vi "SVT Initialize Swept Sine (DAQmx) (1 AO, 2 AI).vi"(8 "error in (no error)":errorcluster, 9 "AI response settings":T5={"response channel"="", "max value [V]"=10.0, "min value [V]"=-10.0, "terminal configuration"=-1} {"terminal configuration" items=["Default"=-1, "RSE"=10083, "NRSE"=10078, "Differential"=10106, "Pseudodifferential"=12529]; "min value [V]" format="%.2f"; "max value [V]" format="%.2f"}, 10 "AI stimulus settings":T6={"stimulus channel"="", "max value [V]"=10.0, "min value [V]"=-10.0, "terminal configuration"=-1} {"terminal configuration" items=["Default"=-1, "RSE"=10083, "NRSE"=10078, "Differential"=10106, "Pseudodifferential"=12529]; "min value [V]" format="%.2f"; "max value [V]" format="%.2f"}, 11 "AO source settings":T7={"excitation channel"="", "max value [V]"=10.0, "min value [V]"=-10.0, "terminal configuration"=-1} {"terminal configuration" items=["Default"=-1, "RSE"=10083, "Differential"=10106, "Pseudodifferential"=12529]; "min value [V]" format="%0.2f"; "max value [V]" format="%0.2f"}) -> (0 "error out":errorcluster, 3 "swept sine task out":T1={"source settings"={"AO task name"="", "source"=[]}, "stimulus settings"={"stimulus task name"="", "stimulus"=[]}, "response(s) settings"={"response task name"="", "response"=[]}, "measurement settings"={"AI sampling frequency"=51200.0, "AO sampling frequency"=1024.0, "AI block size"=1024, "AO block Size"=1024, "block duration [ms]"=0.0, "number of AI channels"=0, "device propagation delay [samples]"=0.0, "total propagation time [samples]"=0.0, "DUT propagation time [ms]"=0.0}, "linlog"=enum."linear", "repeat"=enum."off", "frequency list"=[1.0], "amplitude list"=[1.0], "settling time"={"settle time"=0.015599999576807022, "settle cycles"=5}, "integration time"={"integration time"=0.015599999576807022, "integration cycles"=5}, "frequencies indices"={"AI freq index"=0, "AO freq index"=5}, "read marks"={"write index"=0, "read index"=0, "freq start index"=0, "freq stop index"=0, "# extracted"=0, "buffer type"=enum."Invalid buffer", "read/write indices"=[], "AO index"=0, "AI index"=0, "settled"=FALSE, "integration done"=FALSE}, "harmonic settings"={"maximum THD harmonic"=5, "harmonic mapping"=[1], "units"={"THD unit"=enum."%", "nth harmonic unit"=enum."%", "SINAD unit"=enum."dB", "THD+N unit"=enum."dB"}}, "auto resolution settings"={"auto max step"=512, "slow threshold db"=6.0, "fast threshold db"=1.0}, "auto level settings"={"auto level enable"=FALSE, "auto level channel"=6, "ideal ref"=1.0, "max level"=10.0, "ref upper deviation db"=3.0, "ref lower deviation db"=-3.0}, "offset"=1.0, "ramping rate"=0.0, "phase"=0.0, "initialize"=FALSE} {"phase" format="%.2f"; "response(s) settings"."response"."channel info"."pregain" format="%.2f"; "response(s) settings"."response"."channel info"."weighting filter" items=["Linear", "A-weighting", "B-weighting", "C-weighting", "ITU-R 468-4", "Dolby", "CCITT", "C-message", "Wb", "Wc", "Wd", "We", "Wf", "Wh", "Wj", "Wk", "Wm", "AES17 20 kHz lowpass", "AES17 40 kHz lowpass", "AES17 20 kHz highpass", "AES17 40 kHz highpass"]; "response(s) settings"."response"."channel info"."dB reference" format="%^.1e"; "response(s) settings"."response"."channel info"."engineering units" items=["custom..."=0, "V"=1, "A"=21, "C"=30, "pC"=31, "s"=32, "-"=29, "Pa"=2, "N"=20, "g"=3, "m/s^2"=4, "m/s"=5, "m"=6, "mm/s"=12, "mm"=13, "micron/s"=14, "micron"=15, "in/s^2"=7, "in/s"=8, "in"=9, "mil/s"=10, "mil"=11, "rad/s^2"=16, "rad/s"=17, "rad"=18, "deg/s^2"=26, "deg/s"=27, "deg"=28, "RPM"=22, "cycle/s^2"=23, "Hz"=24, "cycle"=25, "strain"=19]; "response(s) settings"."response"."channel info"."sensor sensitivity" format="%#_5f"; "stimulus settings"."stimulus"."channel info"."pregain" format="%.2f"; "stimulus settings"."stimulus"."channel info"."weighting filter" items=["Linear", "A-weighting", "B-weighting", "C-weighting", "ITU-R 468-4", "Dolby", "CCITT", "C-message", "Wb", "Wc", "Wd", "We", "Wf", "Wh", "Wj", "Wk", "Wm", "AES17 20 kHz lowpass", "AES17 40 kHz lowpass", "AES17 20 kHz highpass", "AES17 40 kHz highpass"]; "stimulus settings"."stimulus"."channel info"."dB reference" format="%^.1e"; "stimulus settings"."stimulus"."channel info"."engineering units" items=["custom..."=0, "V"=1, "A"=21, "C"=30, "pC"=31, "s"=32, "-"=29, "Pa"=2, "N"=20, "g"=3, "m/s^2"=4, "m/s"=5, "m"=6, "mm/s"=12, "mm"=13, "micron/s"=14, "micron"=15, "in/s^2"=7, "in/s"=8, "in"=9, "mil/s"=10, "mil"=11, "rad/s^2"=16, "rad/s"=17, "rad"=18, "deg/s^2"=26, "deg/s"=27, "deg"=28, "RPM"=22, "cycle/s^2"=23, "Hz"=24, "cycle"=25, "strain"=19]; "stimulus settings"."stimulus"."channel info"."sensor sensitivity" format="%#_5f"; "ramping rate" format="%.4f"; "offset" format="%.2f"; "auto level settings"."ref lower deviation db" format="%.4f"; "auto level settings"."ref upper deviation db" format="%.4f"; "auto level settings"."max level" format="%.4f"; "auto level settings"."ideal ref" format="%.4f"; "auto resolution settings"."fast threshold db" format="%.4f"; "auto resolution settings"."slow threshold db" format="%.4f"; "harmonic settings"."maximum THD harmonic" max=10 step=1; "integration time"."integration time" format="%.2p"; "settling time"."settle time" format="%.2p"; "amplitude list" format="%.2f"; "frequency list" format="%.2f"; "measurement settings"."DUT propagation time [ms]" format="%.2f"; "measurement settings"."AO sampling frequency" format="%.2f"; "measurement settings"."AI sampling frequency" format="%.2f"})   [LabVIEW 2017, in "SoundVib_SweptSine.lvlib"]
doc: "Initializes swept-sine-analysis parameters on analog input and output devices."
uses:
  <vilib>/addons/Sound and Vibration/svt_Swept Sine/SoundVib_SweptSine.lvlib
  <vilib>/addons/Sound and Vibration/svt_Swept Sine/subVIs/sv_Swept Sine Task.ctl
  <vilib>/addons/_NISVFA/_Shared subVIs/Controls/svc_Channel Info.ctl
  <vilib>/addons/_NISVFA/_Shared subVIs/Controls/svc_Engineering Units Text Ring.ctl
  <vilib>/addons/_NISVFA/_Shared subVIs/Controls/svc_Weighting Filter Text Ring.ctl
  <vilib>/DAQmx/create/channels.llb/DAQmx Create Channel (AI-Voltage-Basic).vi
  <vilib>/DAQmx/create/channels.llb/DAQmx Create Channel (AO-Voltage-Basic).vi
  <resource>/objmgr/daqmx.rc
panel:
  in  "swept sine task default":T1={"source settings"={"AO task name"="", "source"=[]}, "stimulus settings"={"stimulus task name"="", "stimulus"=[]}, "response(s) settings"={"response task name"="", "response"=[]}, "measurement settings"={"AI sampling frequency"=51200.0, "AO sampling frequency"=51200.0, "AI block size"=1024, "AO block Size"=0, "block duration [ms]"=1024.0, "number of AI channels"=0, "device propagation delay [samples]"=0.0, "total propagation time [samples]"=0.0, "DUT propagation time [ms]"=0.0}, "linlog"=enum."linear", "repeat"=enum."off", "frequency list"=[1.0], "amplitude list"=[1.0], "settling time"={"settle time"=0.015599999576807022, "settle cycles"=5}, "integration time"={"integration time"=0.015599999576807022, "integration cycles"=5}, "frequencies indices"={"AI freq index"=0, "AO freq index"=0}, "read marks"={"write index"=0, "read index"=0, "freq start index"=0, "freq stop index"=0, "# extracted"=0, "buffer type"=enum."Invalid buffer", "read/write indices"=[], "AO index"=0, "AI index"=0, "settled"=FALSE, "integration done"=FALSE}, "harmonic settings"={"maximum THD harmonic"=5, "harmonic mapping"=[1], "units"={"THD unit"=enum."%", "nth harmonic unit"=enum."%", "SINAD unit"=enum."dB", "THD+N unit"=enum."dB"}}, "auto resolution settings"={"auto max step"=512, "slow threshold db"=6.0, "fast threshold db"=1.0}, "auto level settings"={"auto level enable"=FALSE, "auto level channel"=0, "ideal ref"=1.0, "max level"=10.0, "ref upper deviation db"=3.0, "ref lower deviation db"=-3.0}, "offset"=1.0, "ramping rate"=0.0, "phase"=0.0, "initialize"=FALSE} {"phase" format="%.2f"; "response(s) settings"."response"."channel info"."pregain" format="%.2f"; "response(s) settings"."response"."channel info"."weighting filter" items=["Linear", "A-weighting", "B-weighting", "C-weighting", "ITU-R 468-4", "Dolby", "CCITT", "C-message", "Wb", "Wc", "Wd", "We", "Wf", "Wh", "Wj", "Wk", "Wm", "AES17 20 kHz lowpass", "AES17 40 kHz lowpass", "AES17 20 kHz highpass", "AES17 40 kHz highpass"]; "response(s) settings"."response"."channel info"."dB reference" format="%^.1e"; "response(s) settings"."response"."channel info"."engineering units" items=["custom..."=0, "V"=1, "A"=21, "C"=30, "pC"=31, "s"=32, "-"=29, "Pa"=2, "N"=20, "g"=3, "m/s^2"=4, "m/s"=5, "m"=6, "mm/s"=12, "mm"=13, "micron/s"=14, "micron"=15, "in/s^2"=7, "in/s"=8, "in"=9, "mil/s"=10, "mil"=11, "rad/s^2"=16, "rad/s"=17, "rad"=18, "deg/s^2"=26, "deg/s"=27, "deg"=28, "RPM"=22, "cycle/s^2"=23, "Hz"=24, "cycle"=25, "strain"=19]; "response(s) settings"."response"."channel info"."sensor sensitivity" format="%#_5f"; "stimulus settings"."stimulus"."channel info"."pregain" format="%.2f"; "stimulus settings"."stimulus"."channel info"."weighting filter" items=["Linear", "A-weighting", "B-weighting", "C-weighting", "ITU-R 468-4", "Dolby", "CCITT", "C-message", "Wb", "Wc", "Wd", "We", "Wf", "Wh", "Wj", "Wk", "Wm", "AES17 20 kHz lowpass", "AES17 40 kHz lowpass", "AES17 20 kHz highpass", "AES17 40 kHz highpass"]; "stimulus settings"."stimulus"."channel info"."dB reference" format="%^.1e"; "stimulus settings"."stimulus"."channel info"."engineering units" items=["custom..."=0, "V"=1, "A"=21, "C"=30, "pC"=31, "s"=32, "-"=29, "Pa"=2, "N"=20, "g"=3, "m/s^2"=4, "m/s"=5, "m"=6, "mm/s"=12, "mm"=13, "micron/s"=14, "micron"=15, "in/s^2"=7, "in/s"=8, "in"=9, "mil/s"=10, "mil"=11, "rad/s^2"=16, "rad/s"=17, "rad"=18, "deg/s^2"=26, "deg/s"=27, "deg"=28, "RPM"=22, "cycle/s^2"=23, "Hz"=24, "cycle"=25, "strain"=19]; "stimulus settings"."stimulus"."channel info"."sensor sensitivity" format="%#_5f"; "ramping rate" format="%.4f"; "offset" format="%.2f"; "auto level settings"."ref lower deviation db" format="%.4f"; "auto level settings"."ref upper deviation db" format="%.4f"; "auto level settings"."max level" format="%.4f"; "auto level settings"."ideal ref" format="%.4f"; "auto resolution settings"."fast threshold db" format="%.4f"; "auto resolution settings"."slow threshold db" format="%.4f"; "harmonic settings"."maximum THD harmonic" max=10 step=1; "integration time"."integration time" format="%.2p"; "settling time"."settle time" format="%.2p"; "amplitude list" format="%.2f"; "frequency list" format="%.2f"; "measurement settings"."DUT propagation time [ms]" format="%.2f"; "measurement settings"."AO sampling frequency" format="%.2f"; "measurement settings"."AI sampling frequency" format="%.2f"}
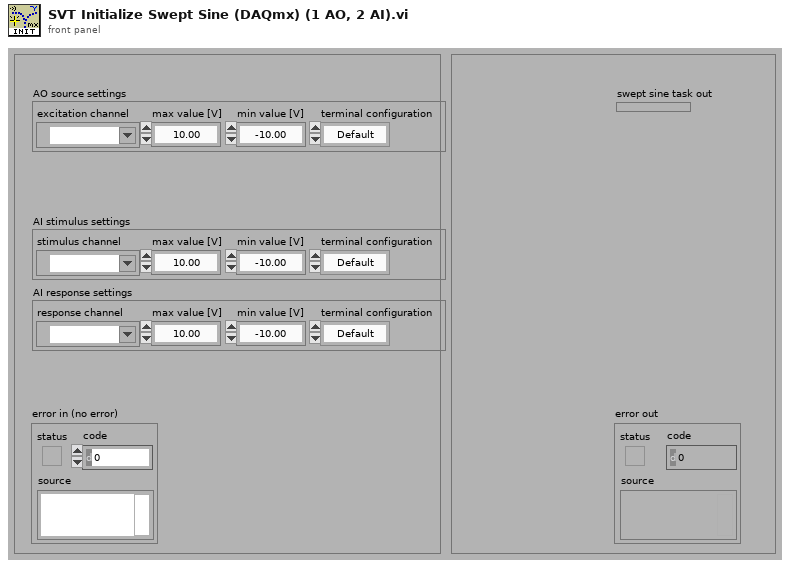
[diagram p1: front panel]
types:
  T1 = typedef "SoundVib_SweptSine.lvlib/sv_Swept Sine Task.ctl" = cluster{"source settings":cluster{"AO task name":refnum<k21>, "source":cluster{"AO physical channel":tag}[]}, "stimulus settings":cluster{"stimulus task name":refnum<k21>, "stimulus":cluster{"stimulus physical channel":tag, "channel info":T2}[]}, "response(s) settings":cluster{"response task name":refnum<k21>, "response":cluster{"response physical channel":tag, "channel info":T2}[]}, "measurement settings":cluster{"AI sampling frequency":dbl, "AO sampling frequency":dbl, "AI block size":i32, "AO block Size":i32, "block duration [ms]":dbl, "number of AI channels":i32, "device propagation delay [samples]":dbl, "total propagation time [samples]":dbl, "DUT propagation time [ms]":dbl}, "linlog":enum16{"linear", "log"}, "repeat":enum16{"off", "on"}, "frequency list":dbl[], "amplitude list":dbl[], "settling time":cluster{"settle time":dbl, "settle cycles":i32}, "integration time":cluster{"integration time":dbl, "integration cycles":i32}, "frequencies indices":cluster{"AI freq index":i32, "AO freq index":i32}, "read marks":cluster{"write index":u32, "read index":u32, "freq start index":u32, "freq stop index":u32, "# extracted":u32, "buffer type":enum16{"Invalid buffer", "Intermediate buffer", "Final buffer"}, "read/write indices":cluster{"settle time index":u32, "integration time index":u32}[], "AO index":i32, "AI index":i32, "settled":bool, "integration done":bool}, "harmonic settings":cluster{"maximum THD harmonic":u32, "harmonic mapping":u32[], "units":cluster{"THD unit":enum16{"dB", "%"}, "nth harmonic unit":enum16{"dB", "%"}, "SINAD unit":enum16{"dB", "%"}, "THD+N unit":enum16{"dB", "%"}}}, "auto resolution settings":cluster{"auto max step":i32, "slow threshold db":dbl, "fast threshold db":dbl}, "auto level settings":cluster{"auto level enable":bool, "auto level channel":u8, "ideal ref":sgl, "max level":sgl, "ref upper deviation db":sgl, "ref lower deviation db":sgl}, "offset":dbl, "ramping rate":dbl, "phase":dbl, "initialize":bool}
  T2 = typedef "svc_Channel Info.ctl" = cluster{"sensor sensitivity":dbl, "engineering units":T3, "dB reference":dbl, "custom label":string, "weighting filter":T4, "pregain":dbl}
  T3 = typedef "svc_Engineering Units Text Ring.ctl" = u16
  T4 = typedef "svc_Weighting Filter Text Ring.ctl" = u16
  T5 = cluster{"response channel":tag, "max value [V]":dbl, "min value [V]":dbl, "terminal configuration":i32}
  T6 = cluster{"stimulus channel":tag, "max value [V]":dbl, "min value [V]":dbl, "terminal configuration":i32}
  T7 = cluster{"excitation channel":tag, "max value [V]":dbl, "min value [V]":dbl, "terminal configuration":i32}
  T8 = cluster{"settle time index":u32, "integration time index":u32}[]
  T9 = enum16{"Invalid buffer", "Intermediate buffer", "Final buffer"}
  T10 = cluster{"DAQmx Physical Channel":tag, "channel info":T2}
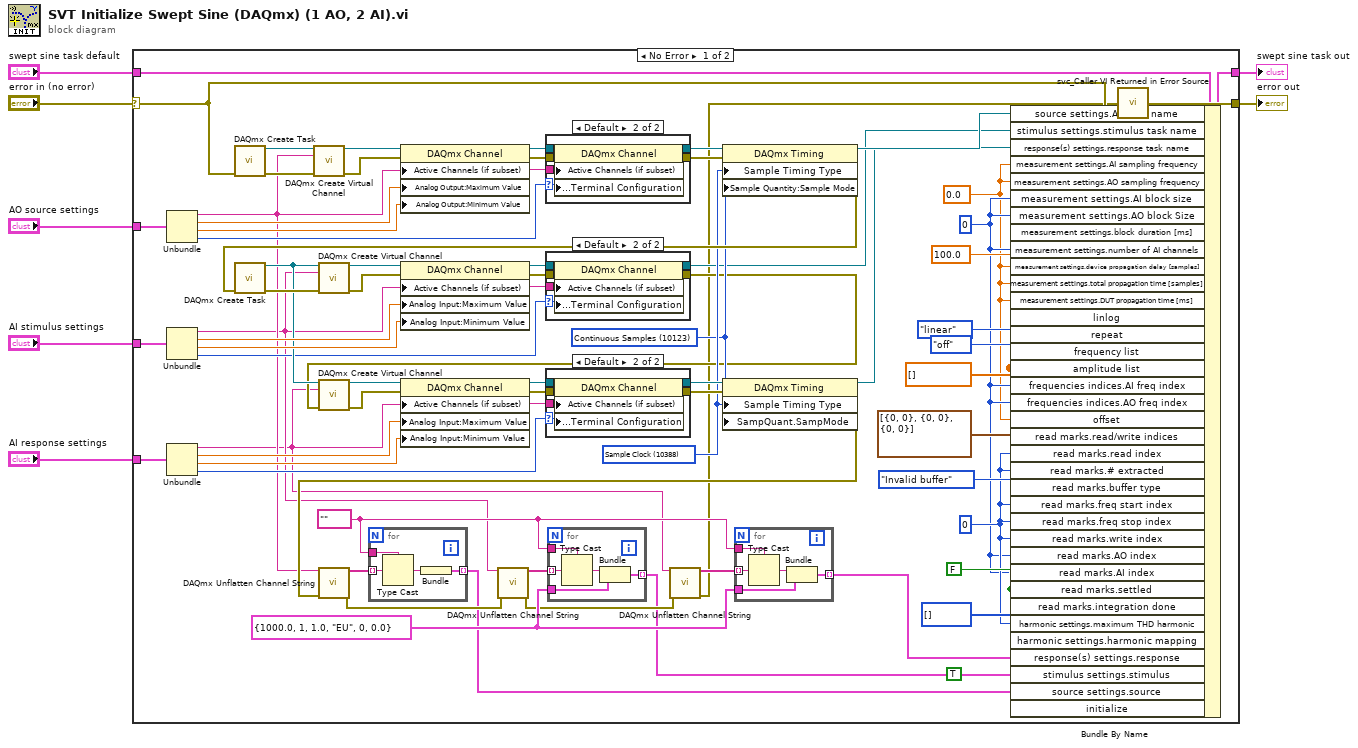
[diagram p0: block diagram]
diagram:
  n1 = case shown="No Error" "error in (no error)" {
    selector: "error in (no error)" -> [w15 w117]
    tunnel: [w70 w117] -> w6
    tunnel: [w67 w116] -> w5
    tunnel: "AO source settings" -> [w55 _]
    tunnel: "AI stimulus settings" -> [w62 _]
    tunnel: "AI response settings" -> [w58 _]
    tunnel: "swept sine task default" -> [w69 w116]
    frame No Error {
      w46 = T2 {"sensor sensitivity"=1000.0, "engineering units"=1, "dB reference"=1.0, "custom label"="EU", "weighting filter"=0, "pregain"=0.0} ("channel info")
      w75 = dbl[] [] ("frequency list")
      w35 = 0.0 ("measurement settings.AI sampling frequency")
      w14 = 10123 items=["Finite Samples"=10178, "Continuous Samples"=10123, "Hardware Timed Single Point"=12522] ("SampQuant.SampMode")
      w17 = 10388 items=["Sample Clock"=10388, "Handshake"=10389, "Implicit"=10451, "On Demand"=10390, "Change Detection"=12504] ("SampTimingType")
      w39 = 0 ("AO device settings.AO Settings.AO taskID")
      w43 = tag "" ("DAQmx Physical Channel")
      w73 = FALSE ("acq state.settled")
      w68 = u32 0 ("AO device settings.AO Settings.AO taskID")
      n2 = Unbundle(w55) -> ("excitation channel"=w10:tag, "max value [V]"=w52:dbl, "min value [V]"=w51:dbl, "terminal configuration"=w28:i32)
      n3 = Unbundle(w62) -> ("stimulus channel"=w9:tag, "max value [V]"=w57:dbl, "min value [V]"=w63:dbl, "terminal configuration"=w27:i32)
      n4 = Unbundle(w58) -> ("response channel"=w8:tag, "max value [V]"=w56:dbl, "min value [V]"=w61:dbl, "terminal configuration"=w26:i32)
      n5 = call <vilib>:"DAQmx Create Task.vi"("error in"=w15) -> ("task out"=w66:refnum<k21>, "error out"=w45:errorcluster)  [unwired: 13 in]
      n6 = call-poly <vilib>:"DAQmx Create Virtual Channel.vi"("task in"=w66, "physical channels"=w10, "error in"=w45) -> ("task out"=w54:refnum<k21>, "error out"=w53:errorcluster)  [unwired: 11 in]
      n7 = property class="DAQmx Channel"(reference=w54, error in=w53, "Active Channels (if subset)"=w10, "Analog Output:Maximum Value"=w52, "Analog Output:Minimum Value"=w51) -> (reference out=w34:refnum<k21>, error out=w33:errorcluster)
      n8 = case shown="Default" w28 {
        selector: w28 -> [_ w96]
        tunnel: w34 -> [w95 w101]
        tunnel: w33 -> [w94 w100]
        tunnel: [w95 w99] -> w24
        tunnel: w10 -> [_ w98]
        tunnel: [w94 w97] -> w20
        frame -1 {
          # "Use default:\nterminal config"
        }
        frame Default {
          n9 = property class="DAQmx Channel"(reference=w101, error in=w100, "Active Channels (if subset)"=w98, "Analog Output:General Properties:Output Configuration:Terminal Configuration"=w96) -> (reference out=w99:refnum<k21>, error out=w97:errorcluster)
        }
      }
      n10 = property class="DAQmx Timing"(reference=w24, error in=w20, "Sample Timing Type"=w17, "Sample Quantity:Sample Mode"=w14) -> (reference out=w25:refnum<k21>, error out=w21:errorcluster)
      n11 = call <vilib>:"DAQmx Create Task.vi"("error in"=w21) -> ("task out"=w42:refnum<k21>, "error out"=w44:errorcluster)  [unwired: 13 in]
      n12 = call-poly <vilib>:"DAQmx Create Virtual Channel.vi"("task in"=w42, "physical channels"=w9, "error in"=w44) -> ("task out"=w64:refnum<k21>, "error out"=w65:errorcluster)  [unwired: 11 in]
      n13 = property class="DAQmx Channel"(reference=w64, error in=w65, "Active Channels (if subset)"=w9, "Analog Input:Maximum Value"=w57, "Analog Input:Minimum Value"=w63) -> (reference out=w32:refnum<k21>, error out=w31:errorcluster)
      n14 = case shown="Default" w27 {
        selector: w27 -> [_ w88]
        tunnel: w32 -> [w87 w93]
        tunnel: w31 -> [w86 w92]
        tunnel: [w87 w91] -> w12
        tunnel: w9 -> [_ w90]
        tunnel: [w86 w89] -> w13
        frame -1 {
          # "Use default:\nterminal config"
        }
        frame Default {
          n15 = property class="DAQmx Channel"(reference=w93, error in=w92, "Active Channels (if subset)"=w90, "Analog Input:General Properties:Input Configuration:Terminal Configuration"=w88) -> (reference out=w91:refnum<k21>, error out=w89:errorcluster)
        }
      }
      n16 = call-poly <vilib>:"DAQmx Create Virtual Channel.vi"("task in"=w42, "physical channels"=w8, "error in"=w13) -> ("task out"=w60:refnum<k21>, "error out"=w59:errorcluster)  [unwired: 11 in]
      n17 = property class="DAQmx Channel"(reference=w60, error in=w59, "Active Channels (if subset)"=w8, "Analog Input:Maximum Value"=w56, "Analog Input:Minimum Value"=w61) -> (reference out=w30:refnum<k21>, error out=w29:errorcluster)
      n18 = case shown="Default" w26 {
        selector: w26 -> [_ w80]
        tunnel: w30 -> [w79 w85]
        tunnel: w29 -> [w78 w84]
        tunnel: [w79 w83] -> w22
        tunnel: w8 -> [_ w82]
        tunnel: [w78 w81] -> w18
        frame -1 {
          # "Use default:\nterminal config"
        }
        frame Default {
          n19 = property class="DAQmx Channel"(reference=w85, error in=w84, "Active Channels (if subset)"=w82, "Analog Input:General Properties:Input Configuration:Terminal Configuration"=w80) -> (reference out=w83:refnum<k21>, error out=w81:errorcluster)
        }
      }
      n20 = property class="DAQmx Timing"(reference=w22, error in=w18, "Sample Timing Type"=w17, "SampQuant.SampMode"=w14) -> (reference out=w23:refnum<k21>, error out=w19:errorcluster)
      n21 = call <vilib>:"DAQmx Unflatten Channel String.vi"("names in"=w10, "error in"=w19) -> ("names out"=w50:string[], "error out"=w41:errorcluster)  [unwired: 12 in]
      n22 = for {
        tunnel: w50 -> [w114] mode=indexing
        tunnel: [w115] -> w38 mode=indexing
        tunnel: w43 -> [w112]
        n23 = Type Cast(type=w112, x=w114) -> (*(type *) &x=w113:tag)
        n24 = Bundle("DAQmx Physical Channel"=w113) -> (w115:cluster{"DAQmx Physical Channel":tag})  [unwired: 1 in]
      }
      n25 = call <vilib>:"DAQmx Unflatten Channel String.vi"("names in"=w9, "error in"=w41) -> ("names out"=w49:string[], "error out"=w40:errorcluster)  [unwired: 12 in]
      n26 = for {
        tunnel: w49 -> [w110] mode=indexing
        tunnel: [w111] -> w37 mode=indexing
        tunnel: w43 -> [w108]
        tunnel: w46 -> [w107]
        n27 = Type Cast(type=w108, x=w110) -> (*(type *) &x=w109:tag)
        n28 = Bundle("DAQmx Physical Channel"=w109, "channel info"=w107) -> (w111:T10)  [unwired: 1 in]
      }
      n29 = call <vilib>:"DAQmx Unflatten Channel String.vi"("names in"=w8, "error in"=w40) -> ("names out"=w47:string[], "error out"=w11:errorcluster)  [unwired: 12 in]
      n30 = for {
        tunnel: w47 -> [w105] mode=indexing
        tunnel: [w106] -> w36 mode=indexing
        tunnel: w43 -> [w103]
        tunnel: w46 -> [w102]
        n31 = Type Cast(type=w103, x=w105) -> (*(type *) &x=w104:tag)
        n32 = Bundle("DAQmx Physical Channel"=w104, "channel info"=w102) -> (w106:T10)  [unwired: 1 in]
      }
      n33 = Bundle By Name(cluster=w69, "source settings.AO task name"=w25, "stimulus settings.stimulus task name"=w12, "response(s) settings.response task name"=w23, "measurement settings.AI sampling frequency"=w35, "measurement settings.AO sampling frequency"=w35, "measurement settings.AI block size"=w39, "measurement settings.AO block Size"=w39, "measurement settings.block duration [ms]"=100.0, "measurement settings.number of AI channels"=w39, "measurement settings.device propagation delay [samples]"=w35, "measurement settings.total propagation time [samples]"=w35, "measurement settings.DUT propagation time [ms]"=w35, "linlog"=enum16{"linear", "log"}."linear", "repeat"=enum16{"off", "on"}."off", "frequency list"=w75, "amplitude list"=w75, "frequencies indices.AI freq index"=w39, "frequencies indices.AO freq index"=w39, "offset"=w35, "read marks.read/write indices"=T8 [{"settle time index"=0, "integration time index"=0}, {"settle time index"=0, "integration time index"=0}, {"settle time index"=0, "integration time index"=0}] ("initialized array"), "read marks.read index"=w68, "read marks.# extracted"=w68, "read marks.buffer type"=T9."Invalid buffer", "read marks.freq start index"=w68, "read marks.freq stop index"=w68, "read marks.write index"=w68, "read marks.AO index"=w39, "read marks.AI index"=w39, "read marks.settled"=w73, "read marks.integration done"=w73, "harmonic settings.maximum THD harmonic"=w68, "harmonic settings.harmonic mapping"=u32[] [], "response(s) settings.response"=w36, "stimulus settings.stimulus"=w37, "source settings.source"=w38, "initialize"=TRUE) -> (w67:T1)
      n34 = call <vilib>:"svc_Caller VI Returned in Error Source.vi"("warning input to caller"=w15, "error in (no error)"=w11) -> ("error out"=w70:errorcluster)  [unwired: 3 in]
    }
    frame Error {
    }
  }
  "error out" <- w6
  "swept sine task out" <- w5
